vi "Get Ingredients.vi"(8 "error in (no error)":errorcluster, 11 "Chemicals in":refnum<class "Chemicals.lvclass">) -> (0 "error out":errorcluster, 2 "Ingredients":T1[](array[typedef]), 3 "Chemicals out":refnum<class "Chemicals.lvclass">)   [LabVIEW 2020, in "Chemicals.lvclass"]
uses:
  Chemicals.lvclass
  Item/Ingredient.ctl
  Item/Item.lvclass
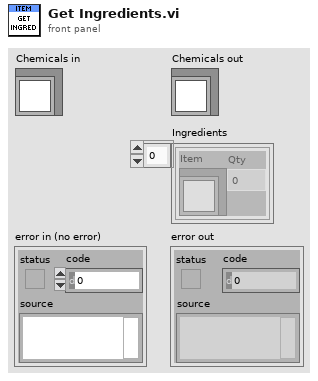
[diagram p1: front panel]
types:
  T1 = typedef "Item.lvclass/Ingredient.ctl" = cluster{"Item":refnum<class "Item.lvclass">, "Qty":dbl}
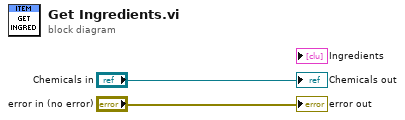
[diagram p0: block diagram]
diagram:
  "error out" <- "error in (no error)"
  "Chemicals out" <- "Chemicals in"
